vi "Locate Installed VIDoc Editors.vi"(8 "Error in":errorcluster caption="Error in (no error)", 11 "VIDoc Settings Directory":path) -> (0 "Error out":errorcluster, 3 "VIDoc Editors":refnum<class "VIDoc Settings.lvclass">[](array[class]))   [LabVIEW 2023]
doc: "Looks for an loads all VIDoc Editors in the <vilib>/DMC/VIDoc/Printers folder.\n\nOptional input to allow calling from an implimentation for testing purposes."
uses:
  Settings/VIDoc Settings/VIDoc Settings.lvclass
  <vilib>/Utility/Symbolic Paths/NI_SymbolicPaths.lvlib
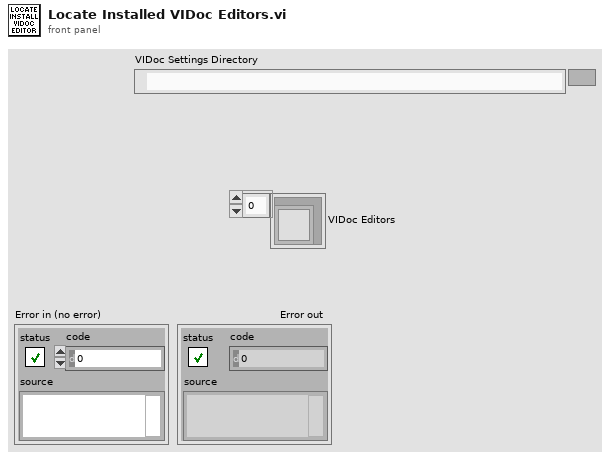
[diagram p1: front panel]
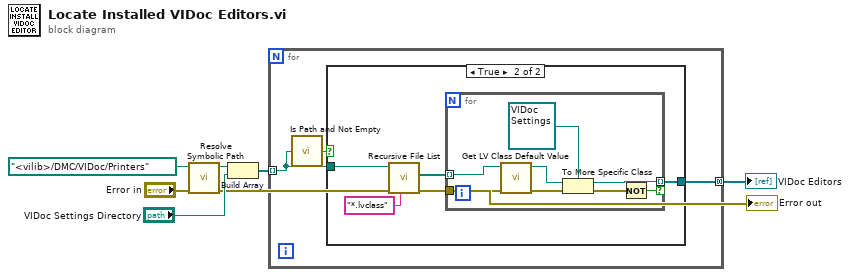
[diagram p0: block diagram]
diagram:
  n1 = call <vilib>:"Resolve Symbolic Path.vi"("error in"="Error in", "path"=path "<vilib>/DMC/VIDoc/Printers") -> ("error out"=→"Error out":errorcluster, "resolved path"=w4:path)  [unwired: 7 in, 1 out]
  n2 = Build Array(w4, "VIDoc Settings Directory") -> (w3:path[])
  n3 = for {
    tunnel: [w10] -> w7 mode=concatenating
    tunnel: w3 -> [w8] mode=indexing
    n4 = call <vilib>:"Is Path and Not Empty.vi"("path"=w8) -> ("Is Path and Not Empty?"=w9:bool)  [unwired: 4 in]
    n5 = case shown="True" w9 {
      tunnel: [_ w12] -> w10
      tunnel: w8 -> [_ w11]
      frame False {
      }
      frame True {
        n6 = call <vilib>:"Recursive File List.vi"("pattern"="*.lvclass", "Folder Path"=w11) -> ("error out"=w13:errorcluster, "All Files in Dir"=w14:path[])  [unwired: 5 in, 3 out]
        n7 = for {
          tunnel: w14 -> [w22] mode=indexing
          tunnel: [w18] -> w12 mode=indexing if=w16
          tunnel: w13 -> [w23]
          n8 = call <vilib>:"Get LV Class Default Value.vi"("error in (no error)"=w23, "class path"=w22) -> ("error out"=w21:errorcluster, "object"=w20:refnum<class>)  [unwired: 8 in]
          n9 = To More Specific Class(target class=refnum<class "VIDoc Settings.lvclass"> refnum ("VIDoc Settings"), reference=w20, error in=w21) -> (specific class reference=w18:refnum<class "VIDoc Settings.lvclass">, error out=w17:errorcluster)
          n10 = Not(x=w17) -> (.not. x?=w16:bool)
        }
      }
    }
  }
  "VIDoc Editors" <- w7
